vi "Get Employee Names and Types.vi"(8 "错误输入（无错误）":errorcluster, 11 "Employee Info":T1) -> (0 "错误输出":errorcluster, 2 "Colomn Types":variant[](array[variant]), 3 "Column Names":string[](array[string]))   [LabVIEW 2012, in "Employee Info.lvlib"]
uses:
  Employee Info.lvlib
  Employee Info.ctl
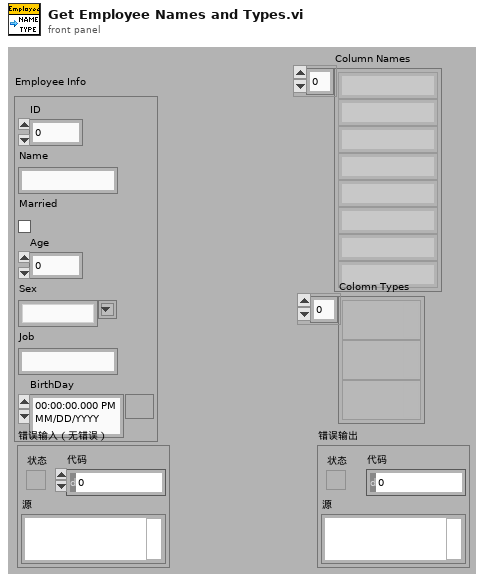
[diagram p1: front panel]
types:
  T1 = typedef "Employee Info.lvlib/Employee Info.ctl" = cluster{"ID":u16, "Name":string, "Married":bool, "Age":u8, "Sex":string, "Job":string, "BirthDay":timestamp}
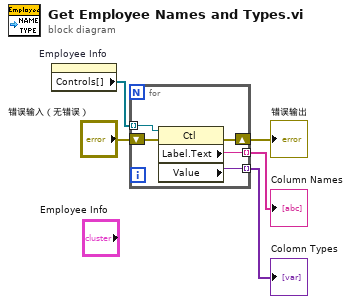
[diagram p0: block diagram]
diagram:
  n1 = property on="Employee Info" class="Clust (严格)"() -> ("Controls[]"=w5:refnum<vi>[])  [unwired: 2 in, 2 out]
  n2 = for {
    tunnel: w5 -> [w10] mode=indexing
    tunnel: [w9] -> w4 mode=indexing
    tunnel: [w8] -> w3 mode=indexing
    shift-right: [w6] -> w1
    shift-left: "错误输入（无错误）" -> [w7]
    n3 = property class="Ctl"(reference=w10, error in=w7) -> (error out=w6:errorcluster, "Label.Text"=w9:string, "Value"=w8:variant)  [unwired: 1 out]
  }
  "Column Names" <- w4
  "Colomn Types" <- w3
  "错误输出" <- w1
